vi "Get Previous Status.vi"(8 "error in (no error)":errorcluster, 11 "abs_Parallel in":refnum<class "abs_Parallel.lvclass">) -> (0 "error out":errorcluster, 2 "Previous Status":T1, 3 "abs_Parallel out":refnum<class "abs_Parallel.lvclass">)   [LabVIEW 2021, in "BT.lvlib" / "abs_Parallel.lvclass"]
uses:
  abs_Parallel.lvclass
  C:/Users/Tim/Documents/GitHub/LV_Behaviour_Tree/Source/abs_Composite/abs_Composite.lvclass
  abs_Node/Status.ctl
  abs_Composite/abs_Composite.lvclass/abs_Composite.ctl
  abs_Parallel.lvclass/abs_Parallel.ctl
  abs_Composite/Properties/Read Index.vi
  abs_Node/abs_Node.lvclass
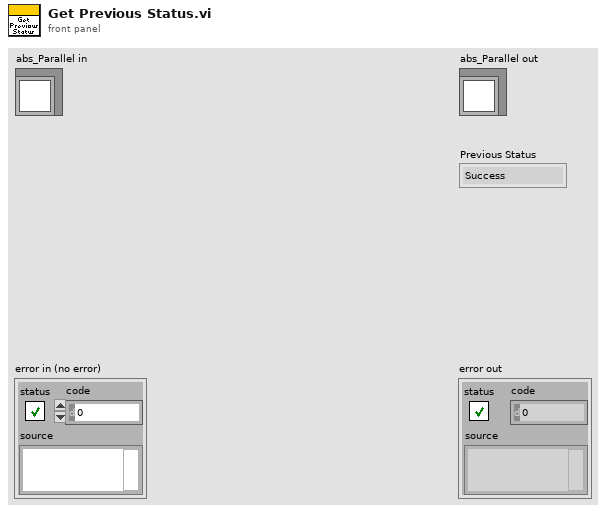
[diagram p1: front panel]
types:
  T1 = typedef "BT.lvlib/abs_Node.lvclass/Status.ctl" = enum16{"Success", "Failure", "Running"}
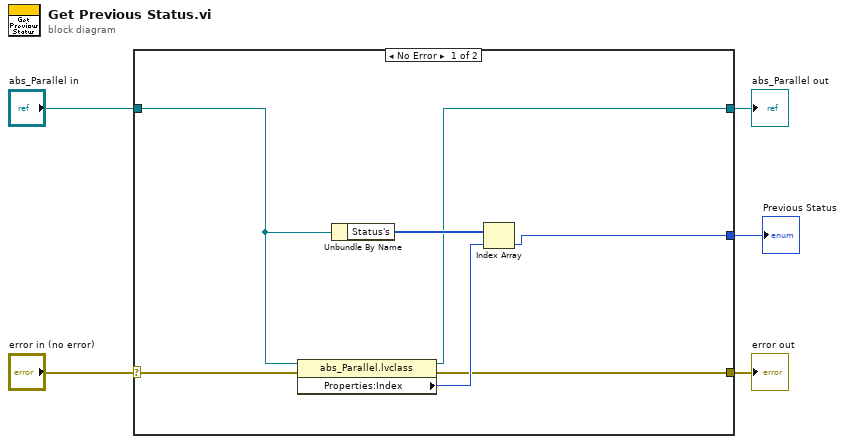
[diagram p0: block diagram]
diagram:
  n1 = case shown="No Error" "error in (no error)" {
    selector: "error in (no error)" -> [w9 w14]
    tunnel: [w8 w14] -> w4
    tunnel: [w7 w13] -> w2
    tunnel: "abs_Parallel in" -> [w10 w13]
    tunnel: [w6 _] -> w1
    frame No Error {
      n2 = property class="abs_Parallel.lvclass"(reference=w10, error in=w9) -> (reference out=w7:refnum<class "abs_Parallel.lvclass">, error out=w8:errorcluster, "Properties:Index"=w11:i32)
      n3 = Unbundle By Name(w10) -> ("Status's"=w12:T1[])
      n4 = Index Array(array=w12, index=w11) -> (element=w6:T1)
    }
    frame Error {
    }
  }
  "error out" <- w4
  "abs_Parallel out" <- w2
  "Previous Status" <- w1
